vi "Mixing.vi"(6 "Mixed Track":path, 8 "Track 2 Volume":i8(slide) scale=0.0..10.0, 9 "Track 2":path, 10 "Track 1 Volume":i8(slide) scale=0.0..10.0, 11 "Track 1":path) -> (0 "Mixed Track":waveform(dbl)(graph), 2 "Track 2":waveform(dbl)(graph), 3 "Track 1":waveform(dbl)(graph))   [LabVIEW 2014]
uses:
  <vilib>/Waveform/WDTFileIO.llb/Read Waveform from File.vi
  <vilib>/Waveform/WDTFileIO.llb/ Write Waveform to File.vi
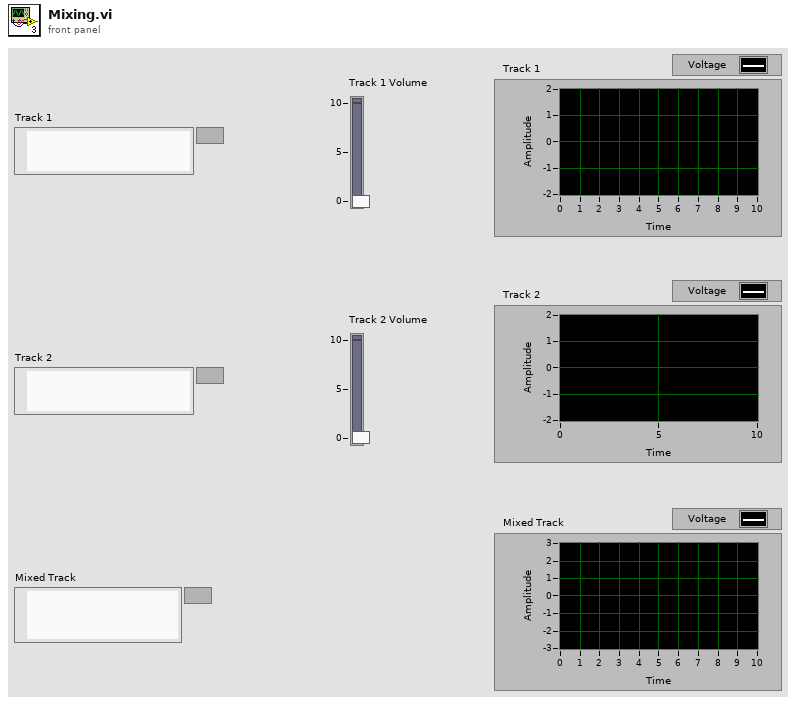
[diagram p1: front panel]
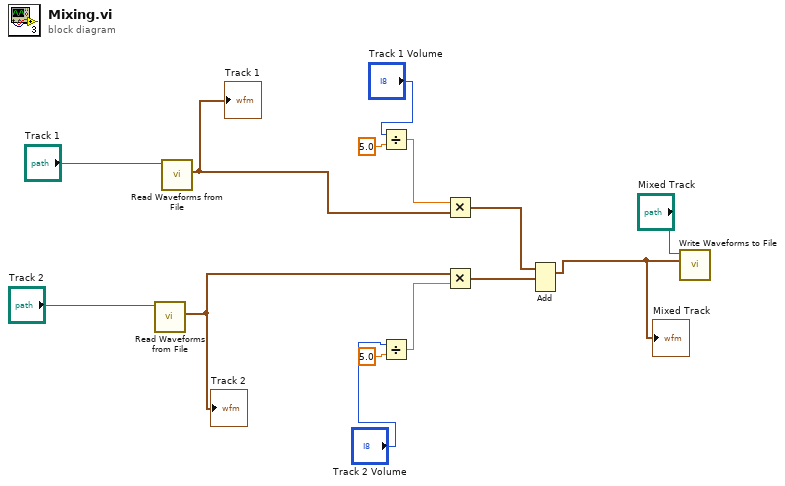
[diagram p0: block diagram]
diagram:
  n1 = call-poly <vilib>:"Read Waveforms from File.vi"("file path (dialog if empty)"="Track 2") -> ("first waveform in record"=w2:waveform(dbl))  [unwired: 5 in, 3 out]
  "Track 2" <- w2
  n2 = call-poly <vilib>:"Read Waveforms from File.vi"("file path (dialog if empty)"="Track 1") -> ("first waveform in record"=w3:waveform(dbl))  [unwired: 5 in, 3 out]
  "Track 1" <- w3
  n3 = Divide(x="Track 1 Volume", y=5.0) -> (x/y=w11:dbl)
  n4 = Divide(x="Track 2 Volume", y=5.0) -> (x/y=w9:dbl)
  n5 = Multiply(x=w11, y=w3) -> (x*y=w7:waveform(dbl))
  n6 = Multiply(x=w2, y=w9) -> (x*y=w8:waveform(dbl))
  n7 = Add(1:w8, 2:w7) -> (0:w1:waveform(dbl))  [unwired: 1 in, 1 out]
  "Mixed Track" <- w1
  n8 = call-poly <vilib>:"Write Waveforms to File.vi"("waveform"=w1, "file path (dialog if empty)"="Mixed Track") -> ()  [unwired: 8 in, 2 out]
